vi "Find Exact Peak.vi"(0 "window":T1(ring)=enum."7 Term B-Harris", 1 "Freq. Resolution":dbl=1e-08 format="%.2e", 2 "Size of FFT (N)":i32=1024 min=0 step=1, 3 "A0":dbl=3.738613052908998e-10 format="%.8f", 4 "A1":dbl=3.686220325397741e-10 format="%.8f") -> (5 "A exact":dbl=3.926212591970866e-10 format="%.8f", 6 "f exact":dbl format="%.8f")   [LabVIEW 2021]
doc: "Finds an accurate approximation to the peak reponse and frequency location using the window coefficients and a binary search algorithm. The best guess is initialized to the center of the frequency bins and is moved within the search loop until the window reponses at the bin edges closely approximate the observed magnitude responses of the original spectrum."
panel:
  in  "max iterations":i32=100 min=0 step=1
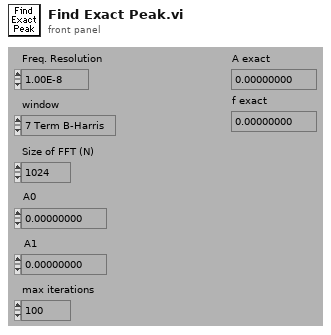
[diagram p1: front panel]
types:
  T1 = enum32{"None ", "Hanning", "Hamming", "Blackman-Harris", "Exact Blackman", "Blackman", "Flat Top", "4 Term B-Harris ", "7 Term B-Harris"}
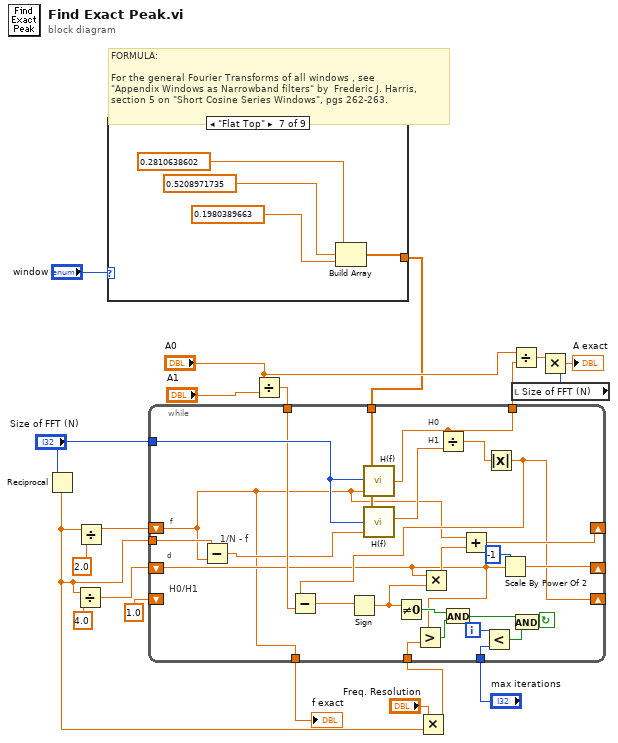
[diagram p0: block diagram]
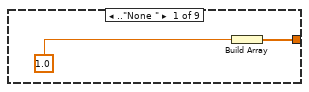
[diagram p2: hidden frame]
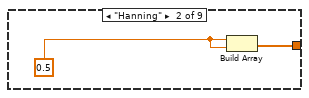
[diagram p3: hidden frame]
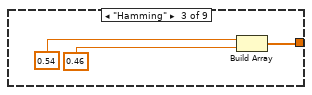
[diagram p4: hidden frame]
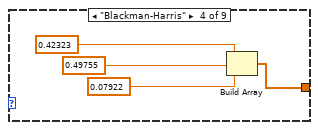
[diagram p5: hidden frame]
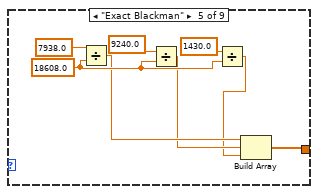
[diagram p6: hidden frame]
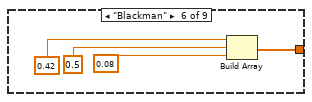
[diagram p7: hidden frame]
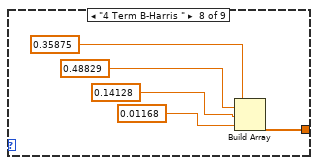
[diagram p8: hidden frame]
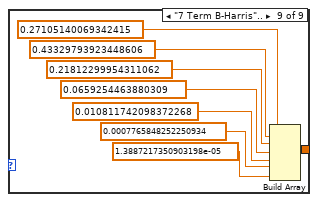
[diagram p9: hidden frame]
diagram:
  # "FORMULA: \n\nFor the general Fourier Transforms of all windows , see \n\"Appendix Windows as Narrowband filters\" by  Frederic J. Harris,\nsection 5 on \"Short Cosine Series Windows\", pgs 262-263."
  n1 = Reciprocal(x="Size of FFT (N)") -> (1/x=w3:dbl)
  n2 = Divide(x=w3, y=4.0) -> (x/y=w14:dbl)
  n3 = Divide(x=w3, y=2.0) -> (x/y=w16:dbl)
  n4 = case shown="\"Flat Top\"" "window" {
    tunnel: [w21 w24 w25 w28 w35 w40 w44 w48 w53] -> w4
    frame .."None " {
      n5 = Build Array(1.0) -> (w21:dbl[])
    }
    frame "Hanning" {
      w23 = 0.5
      n6 = Build Array(w23, w23) -> (w24:dbl[])
    }
    frame "Hamming" {
      n7 = Build Array(0.54, 0.46) -> (w25:dbl[])
    }
    frame "Blackman-Harris" {
      n8 = Build Array(0.42323, 0.49755, 0.07922) -> (w28:dbl[])
    }
    frame "Exact Blackman" {
      w38 = 18608.0
      n9 = Divide(x=7938.0, y=w38) -> (x/y=w34:dbl)
      n10 = Divide(x=9240.0, y=w38) -> (x/y=w33:dbl)
      n11 = Divide(x=1430.0, y=w38) -> (x/y=w32:dbl)
      n12 = Build Array(w34, w33, w32) -> (w35:dbl[])
    }
    frame "Blackman" {
      n13 = Build Array(0.42, 0.5, 0.08) -> (w40:dbl[])
    }
    frame "Flat Top" {
      n14 = Build Array(0.2810638602, 0.5208971735, 0.1980389663) -> (w44:dbl[])
    }
    frame "4 Term B-Harris " {
      n15 = Build Array(0.35875, 0.48829, 0.14128, 0.01168) -> (w48:dbl[])
    }
    frame "7 Term B-Harris".. {
      n16 = Build Array(0.27105140069342415, 0.43329793923448606, 0.21812299954311062, 0.0659254463880309, 0.010811742098372268, 0.0007765848252250934, 1.3887217350903198e-05) -> (w53:dbl[])
    }
  }
  n17 = Divide(x="A0", y="A1") -> (x/y=w6:dbl)
  n18 = Multiply(x="Freq. Resolution", y=w3) -> (x*y=w1:dbl)
  n19 = while {
    tunnel: "max iterations" -> [w65]
    tunnel: w1 -> [w67]
    tunnel: [w63] -> w11
    tunnel: [w61] -> w10
    tunnel: w6 -> [w81]
    shift-left: 1.0 -> [_]
    shift-right: [w74] -> _
    tunnel: w3 -> [w84]
    shift-left: w14 -> [w66]
    shift-right: [w75] -> _
    shift-left: w16 -> [w61]
    shift-right: [w77] -> _
    tunnel: w4 -> [w64]
    tunnel: "Size of FFT (N)" -> [w83]
    i -> [w73]
    stop <- w69 continue-if-true
    # "H0/H1"
    # "d"
    # "1/N - f"
    # "f"
    # "H1"
    # "H0"
    n20 = Subtract(x=w84, y=w61) -> (x-y=w62:dbl)
    n21 = call "H(f).vi"("f"=w61, "N"=w83, "An"=w64) -> ("y"=w63:dbl)
    n22 = call "H(f).vi"("f"=w62, "N"=w83, "An"=w64) -> ("y"=w85:dbl)
    n23 = Greater?(x=w66, y=w67) -> (0:w72:bool)
    n24 = Divide(x=w63, y=w85) -> (x/y=w82:dbl)
    n25 = Less?(x=w73, y=w65) -> (x < y?=w71:bool)
    n26 = Absolute Value(x=w82) -> (abs(x)=w74:dbl)
    n27 = Subtract(x=w74, y=w81) -> (x-y=w68:dbl)
    n28 = Sign(1:w68) -> (0:w79:dbl)
    n29 = Not Equal To 0?(x=w79) -> (x != 0?=w80:bool)
    n30 = Multiply(x=w66, y=w79) -> (x*y=w78:dbl)
    n31 = And(x=w80, y=w72) -> (x .and. y?=w70:bool)
    n32 = Add(x=w61, y=w78) -> (x+y=w77:dbl)
    n33 = Scale By Power Of 2(n=-1, x=w66) -> (x*2^n=w75:dbl)
    n34 = And(x=w70, y=w71) -> (x .and. y?=w69:bool)
  }
  "f exact" <- w10
  n35 = Divide(x="A0", y=w11) -> (x/y=w9:dbl)
  n36 = local read "Size of FFT (N)"() -> (w7:i32)
  n37 = Multiply(x=w9, y=w7) -> (x*y=→"A exact":dbl)
